vi "CMD_Harvest.vi"(1 "Line":string) -> (0 "Done":bool)   [LabVIEW 2016]
uses:
  <vilib>/Rock Robotics/WPI/ThirdParty/CanMotor/TalonSRX/WPI_CANTalonSRX_APIControlMode.ctl
panel:
  in  "Parameters":i32[](array[numeric])=[1, 1, 1, 1]
  in  "Subcommands":string[](array[string])=["motor", "at", "for", "until"]
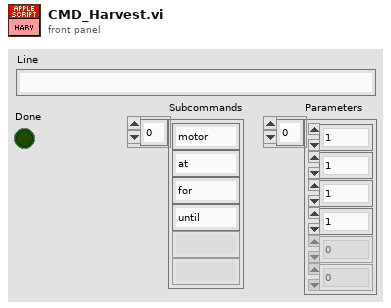
[diagram p1: front panel]
types:
  T1 = typedef "WPI_CANTalonSRX_APIControlMode.ctl" = enum8{"Percent VBus", "Speed", "Position", "Slave", "Unchanged / Invalid", "Voltage Compensation", "Current", "Motion Profile", "Motion Magic"}
  T2 = typedef "WPI_MotorControlDeviceRef.ctl" = cluster{"DeviceStatus":errorcluster, "Type":T3, "PWM":cluster{"PWM Channel":T4, "DeadBand":T5}, "CAN":cluster{"Device Number":u8, "SetOutput VI Ref":variant, "GetOutput VI Ref":variant, "Enable VI Ref":variant, "Disable VI Ref":variant, "Data":variant}, "Invert":bool}
  T3 = typedef "WPI_MotorControlType.ctl" = enum16{"PWM", "CAN"}
  T4 = typedef "FPGA_DIOPWMChannel.ctl" = enum8{"PWM 0", "PWM 1", "PWM 2", "PWM 3", "PWM 4", "PWM 5", "PWM 6", "PWM 7", "PWM 8", "PWM 9", "PWM MXP 0", "PWM MXP 1", "PWM MXP 2", "PWM MXP 3", "PWM MXP 4", "PWM MXP 5", "PWM MXP 6", "PWM MXP 7", "PWM MXP 8", "PWM MXP 9", "Invalid"}
  T5 = typedef "WPI_PWMDeadband.ctl" = cluster{"Name":string, "maxPositivePwm":i32, "minPositivePwm":i32, "centerPwm":i32, "maxNegativePwm":i32, "minNegativePwm":i32, "angularRange":u16}
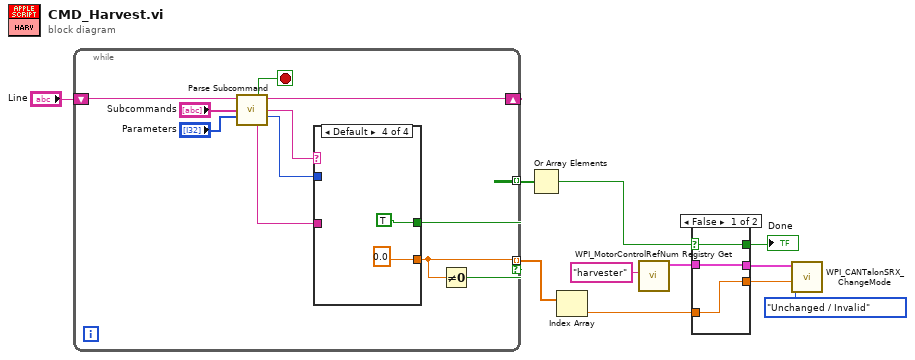
[diagram p0: block diagram]
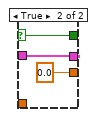
[diagram p2: hidden frame]
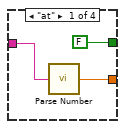
[diagram p3: hidden frame]
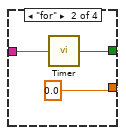
[diagram p4: hidden frame]
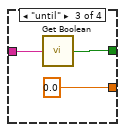
[diagram p5: hidden frame]
diagram:
  n1 = while {
    shift-right: [w19] -> _
    shift-left: "Line" -> [w22]
    tunnel: [w14] -> w10 mode=indexing
    tunnel: [w13] -> w9 mode=indexing if=w12
    stop <- w18 stop-if-true
    n2 = call "Parse Subcommand.vi"("Text In"=w22, "Subcommands"="Subcommands", "Parameters"="Parameters") -> ("Done"=w18:bool, "Text Out"=w19:string, "Subcommand"=w17:string, "# of Parameters"=w16:i32, "Parameter 1"=w15:string)  [unwired: 6 in, 2 out]
    n3 = case shown="Default" w17 {
      tunnel: w16 -> [_ _ _ _]
      tunnel: w15 -> [w25 w28 w31 _]
      tunnel: [FALSE ("Value") w26 w29 TRUE ("Value")] -> w14
      tunnel: [w23 0.0 ("Number") 0.0 ("Number") 0.0 ("Number")] -> w13
      frame "at" {
        n4 = call "Parse Number.vi"("String"=w25) -> ("Number"=w23:dbl)
      }
      frame "for" {
        n5 = call "Timer.vi"("Seconds (string)"=w28) -> ("Done"=w26:bool)
      }
      frame "until" {
        n6 = call "Get Boolean.vi"("Name"=w31) -> ("Value"=w29:bool)
      }
      frame Default {
      }
    }
    n7 = Not Equal To 0?(x=w13) -> (x != 0?=w12:bool)
  }
  n8 = Or Array Elements(Boolean array=w10) -> (logical OR=w8:bool)
  n9 = Index Array(array=w9) -> (element=w4:dbl)  [unwired: 1 in]
  n10 = call <vilib>:"WPI_MotorControlRefNum Registry Get.vi"("refnum name"="harvester") -> ("MotorControlDevRef"=w6:T2)  [unwired: 9 in, 1 out]
  n11 = case shown="False" w8 {
    selector: w8 -> [w36 w39]
    tunnel: [w36 w39] -> w7
    tunnel: w6 -> [w35 w38]
    tunnel: [w35 w38] -> w5
    tunnel: w4 -> [w34 _]
    tunnel: [w34 0.0] -> w3
    frame False {
    }
    frame True {
    }
  }
  "Done" <- w7
  n12 = call <vilib>:"WPI_CANTalonSRX_ChangeMode.vi"("Output"=w3, "Control Mode"=WPI_CANTalonSRX_APIControlMode."Unchanged / Invalid", "CAN Talon SRX Ref"=w5) -> ()  [unwired: 7 in, 2 out]
